vi "pigeon_periodic.vi"   [LabVIEW 2020]
uses:
  <vilib>/Rock Robotics/WPI/ThirdParty/Phoenix-LabVIEW/Pigeon IMU/CTRE_PigeonIMU_GetYPR.vi
  <vilib>/Analysis/NI_AAL_Angle.lvlib
  <vilib>/Analysis/coordinate.llb/Wrap Angle (scalar).vi
  <vilib>/Analysis/coordinate.llb/Angle Range (Degree).ctl
  <vilib>/Analysis/coordinate.llb/Angle Units.ctl
  TitanLib/Lib/TitanLib.lvlib
  globals.vi
types:
  T1 = typedef "NI_AAL_Angle.lvlib/Angle Units.ctl" = i32
  T2 = typedef "NI_AAL_Angle.lvlib/Angle Range (Degree).ctl" = u16
  T3 = typedef "WPI_JoystickDevRef.ctl" = cluster{"Device":T4}
  T4 = typedef "WPI_JoystickDeviceEnum.ctl" = enum16{"USB 0", "USB 1", "USB 2", "USB 3", "USB 4", "USB 5"}
  T5 = typedef "CTRE_PigeonIMU_DeviceRef.ctl" = cluster{"DeviceStatus":errorcluster, "Device Number":u8, "Type":T6, "Device ID":u32, "Handle":u64, "UsageFrame":u32, "Library Path":path}
  T6 = typedef "CTRE_PigeonIMU_ConnectionType.ctl" = u32
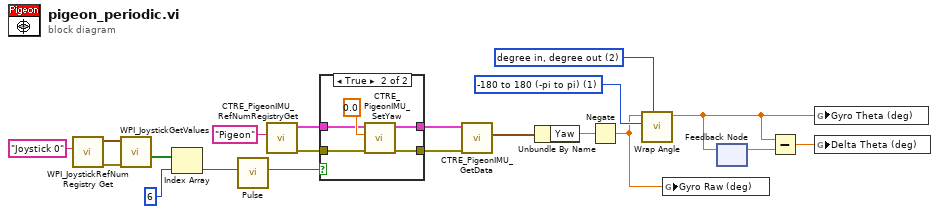
[diagram p0: block diagram]
diagram:
  w16 = T1 2 items=["radian in, radian out", "radian in, degree out", "degree in, degree out", "degree in, radian out"] ("angle units")
  w15 = T2 1 items=["none", "-180 to 180 (-pi to pi)", "0 to 360 (0 to 2pi)"] ("angle range")
  n1 = call <vilib>:"WPI_JoystickRefNum Registry Get.vi"("refnum name"="Joystick 0") -> ("error out"=w9:errorcluster, "JoystickDevRef"=w8:T3)  [unwired: 1 in, 8 out]
  n2 = call <vilib>:"WPI_JoystickGetValues.vi"("error in (no error)"=w9, "JoystickDevRef"=w8) -> ("Buttons"=w6:bool[])  [unwired: 5 in, 4 out]
  n3 = Index Array(array=w6, index=6) -> (element=w4:bool)
  n4 = call "Pulse.vi"("Input"=w4) -> ("Output"=w14:bool)  [unwired: 10 in]
  n5 = call <vilib>:"CTRE_PigeonIMU_RefNumRegistryGet.vi"("refnum name"="Pigeon") -> ("error out"=w1:errorcluster, "PigeonIMUDevRef"=w2:T5)  [unwired: 9 in]
  n6 = case shown="True" w14 {
    tunnel: [w22 w26] -> w18
    tunnel: [w21 w25] -> w19
    tunnel: w2 -> [w22 w24]
    tunnel: w1 -> [w21 w23]
    frame False {
    }
    frame True {
      n7 = call <vilib>:"CTRE_PigeonIMU_SetYaw.vi"("error in (no error)"=w23, "Value"=0.0, "PigeonIMUDevRef"=w24) -> ("error out"=w25:errorcluster, "PigeonIMUDevRef"=w26:T5)  [unwired: 7 in]
    }
  }
  n8 = call-poly <vilib>:"CTRE_PigeonIMU_GetData.vi"("error in (no error)"=w19, "PigeonIMUDevRef"=w18) -> ("Yaw Pitch Roll"=w20:cluster{"Yaw":dbl, "Pitch":dbl, "Roll":dbl})  [unwired: 7 in, 2 out]
  n9 = Unbundle By Name(w20) -> ("Yaw"=w17:dbl)
  n10 = Negate(x=w17) -> (-x=w13:dbl)
  n11 = call-poly <vilib>:"Wrap Angle.vi"("angle units"=w16, "angle range"=w15, "angle in"=w13) -> ("angle out"=w10:dbl)  [unwired: 7 in, 1 out]
  n12 = global write "globals.vi" "Gyro Raw (deg)"(w13) -> ()
  n13 = feedback #1() -> (w11:dbl)  [unwired: 1 in]
  n14 = feedback-in #1(w10) -> ()
  n15 = Subtract(x=w10, y=w11) -> (x-y=w12:dbl)
  n16 = global write "globals.vi" "Gyro Theta (deg)"(w10) -> ()
  n17 = global write "globals.vi" "Delta Theta (deg)"(w12) -> ()
